vi "UIEH(ver.General).vi"() -> ()   [LabVIEW 2023]
panel:
  in  "종료":bool
  in  "저장":bool
  in  "분석":bool
  in  "측정":bool
  out "Count":i32
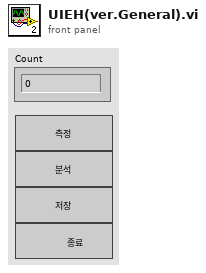
[diagram p1: front panel]
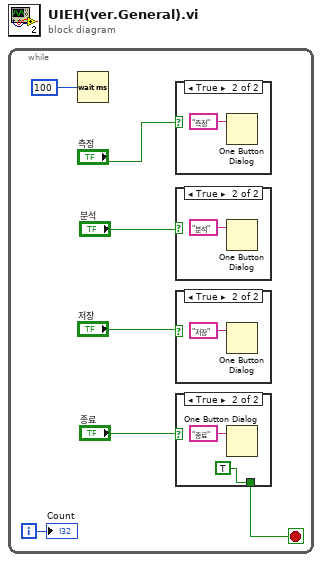
[diagram p0: block diagram]
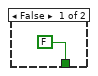
[diagram p2: hidden frame]
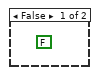
[diagram p3: hidden frame]
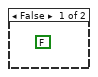
[diagram p4: hidden frame]
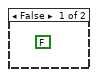
[diagram p5: hidden frame]
diagram:
  n1 = while {
    i -> [w7]
    stop <- w5 stop-if-true
    n2 = Wait (ms)(milliseconds to wait=u32 100) -> ()  [unwired: 1 out]
    n3 = case shown="True" "측정" {
      frame False {
        (unwired) FALSE
      }
      frame True {
        n4 = One Button Dialog(message="측정") -> ()  [unwired: 1 in, 1 out]
      }
    }
    n5 = case shown="True" "분석" {
      frame False {
        (unwired) FALSE
      }
      frame True {
        n6 = One Button Dialog(message="분석") -> ()  [unwired: 1 in, 1 out]
      }
    }
    n7 = case shown="True" "저장" {
      frame False {
        (unwired) FALSE
      }
      frame True {
        n8 = One Button Dialog(message="저장") -> ()  [unwired: 1 in, 1 out]
      }
    }
    n9 = case shown="True" "종료" {
      tunnel: [FALSE TRUE] -> w5
      frame False {
      }
      frame True {
        n10 = One Button Dialog(message="종료") -> ()  [unwired: 1 in, 1 out]
      }
    }
    "Count" <- w7
  }
